vi "2_2_Face_Detection_Eval(FPGA)(PXI,sbRIO_Remote).vi"() -> ()   [LabVIEW 2020]
doc: "This example demonstrates the usage of the \"DeepLTK FPGA Addon\" for deploying a Face Detection model on a PXI-FPGA board, utilizing an input image sourced from a file.\n\nMore Examples: https://github.com/ngenehub/deepltk_fpga_examples"
uses:
  <vilib>/userDefined/High Color/nirio_resource_hc.ctl
  46bc2405-78a8-48b4-9ac8-c57804670a76.vi
  20299fb9-7878-42d1-962c-cdd5eeae2605.vi
  <vilib>/FPGAPlugInAG/Dynamic/niLvFpga_Download_Dynamic.vi
  <vilib>/FPGAPlugInAG/Dynamic/niLvFpga_Run_Dynamic.vi
  <vilib>/Ngene/Deep Learning Toolkit/Toolkit/NN_Data/subVIs/Dataset/NN_Variant_to_DVR/4D/NN_Data_Variant_to_DVR(4D_SGL).vi
  <vilib>/Ngene/Deep Learning Toolkit/Toolkit/NN_Data/subVIs/Get_Data_Vals/4D/NN_Data_Get_ValByRef(4D_SGL_idx).vi
  <vilib>/Ngene/DeepLTK FPGA Addon/Toolkit/NNF_Host/API/NNF_Set_Input/NNF_Set_Input(3D_I8).vi
  <vilib>/Ngene/Deep Learning Toolkit/Toolkit/NN_Train/Eval_Loss/NN_Eval_Test_Error_Loss/NN_Eval(In3D_OutBBox).vi
  <vilib>/Ngene/Deep Learning Toolkit/Toolkit/NN_Train/Eval_Loss/NN_Calc_Cofusion_Matrix/NN_Calc_Confusion_Matrix(In3D_OutBBox).vi
  <vilib>/FPGAPlugInAG/Dynamic/niLvFpga_Close_Dynamic.vi
  <vilib>/rvi/interface/nirviMethod/nirviMethod.xnode
  <vilib>/rvi/interface/nirviCloseFPGA/nirviCloseFPGA.xnode
  <vilib>/Ngene/Deep Learning Toolkit/Toolkit/Deep_Learning_Toolkit_by_Ngene.lvlib
  <vilib>/Ngene/DeepLTK FPGA Addon/Toolkit/DeepLTK_FPGA_Addon.lvlib
  <vilib>/ptbypt/NI_PtbyPt.lvlib
panel:
  out "Eval Time":dbl=0.030917380000028062 format="%#_2p"
  out "Loop time":dbl=0.030853959999512882 format="%#_2p"
  out "Confusion Matrix":string[][](table)=[["26", "6", "0.8125"], ["2", "0", "0.0000"], ["0.9286", "0.0000", ""]]
  out "mAP@0.5":sgl=0.788305
  out "mIOU":sgl=0.59939504
  out "Iterations":i32=19
  out "Dataset Size":i32=20
  in  "Stop":bool
  in  "FPGA Target":T1="rio://10.0.0.39/RIO0" caption="RIO Device"
  in  "FPGA Bitfile":path=path "D:/Ngene/GitHub/deepltk_fpga_examples/FPGA Bitfiles/NNF_sbRIO_9609_8Cores.lvbitx"
  in  "Dataset Path (Annotations)":path=path "D:/Ngene/GitHub/deepltk_fpga_examples/2_Face_Detection(PXI,sbRIO)/Dataset/Annotations"
  in  "Display?":bool
  out "Display":T2(plugin-control)
  in  "Scalers File Path":path=path "D:/Ngene/GitHub/deepltk_fpga_examples/2_Face_Detection(PXI,sbRIO)/Models/Face_Detection_NNF_Converted/NNF_Face_Detection_Scalers.cfg"
  in  "Dataset Path (Images)":path=path "D:/Ngene/GitHub/deepltk_fpga_examples/2_Face_Detection(PXI,sbRIO)/Dataset/Images"
  in  "Confidence_Thresh":sgl=0.46
  in  "IOU_Thresh":sgl=0.4
  in  "Weight File Path":path=path "D:/Ngene/GitHub/deepltk_fpga_examples/2_Face_Detection(PXI,sbRIO)/Models/Face_Detection_NNF_Converted/NNF_Face_Detection.bin"
  in  "Configuration File Path":path=path "D:/Ngene/GitHub/deepltk_fpga_examples/2_Face_Detection(PXI,sbRIO)/Models/Face_Detection_NNF_Converted/NNF_Face_Detection.cfg"
  # "Overview: This VI is designed to evaluate (measure the accuracy of) the model when executed on FPGA in PXI systems.\nThis VI can also be used to run the evaluation on sbRIO Targets remotely (from Windows based PC)\nRequirements: \n• DeepLTK - Deep Learning Toolkit for LabVIEW (https://www.ngene.co/deep-learning-toolkit-for-labview)\n• DeepLTK FPGA Addon (https://www.ngene.co/deepltk-accelerator-for-fpga)\nInstructions:\n1. Select FPGA target at FPGA Target control. PXI or remote sbRIO FPGA target can be specified.\n2. Provide path to compiled FPGA bitfile at FPGA Bitfile control. A sample is available in the \"Examples\\FPGA Bitfiles\" folder. \n3. Provide the path to the dataset to be evaluated at Dataset. A sample is available in the \"Dataset\" folder.\n4. Provide paths to .cfg, .bin and scalers.cfg files generated during model conversion or sample from project (locted in \"Models\\Face_Detection_NNF_Converted\" folder ) at Network Configuration File Path, Weight File Path and Scalers File Path controls.\n5. Run the VI with the default remaining settings.\n6. Observe measured accuracy at mIOU, mAP@0.5 and Confusion Matrix indicator.\n7. Press the Stop button to stop VI.\n7. To measure reference accuracy (when executed on CPU) run 2_1_Face_Detection_Eval(CPU).vi located in the project."
  # "Copy resource path from NI MAX if needed"
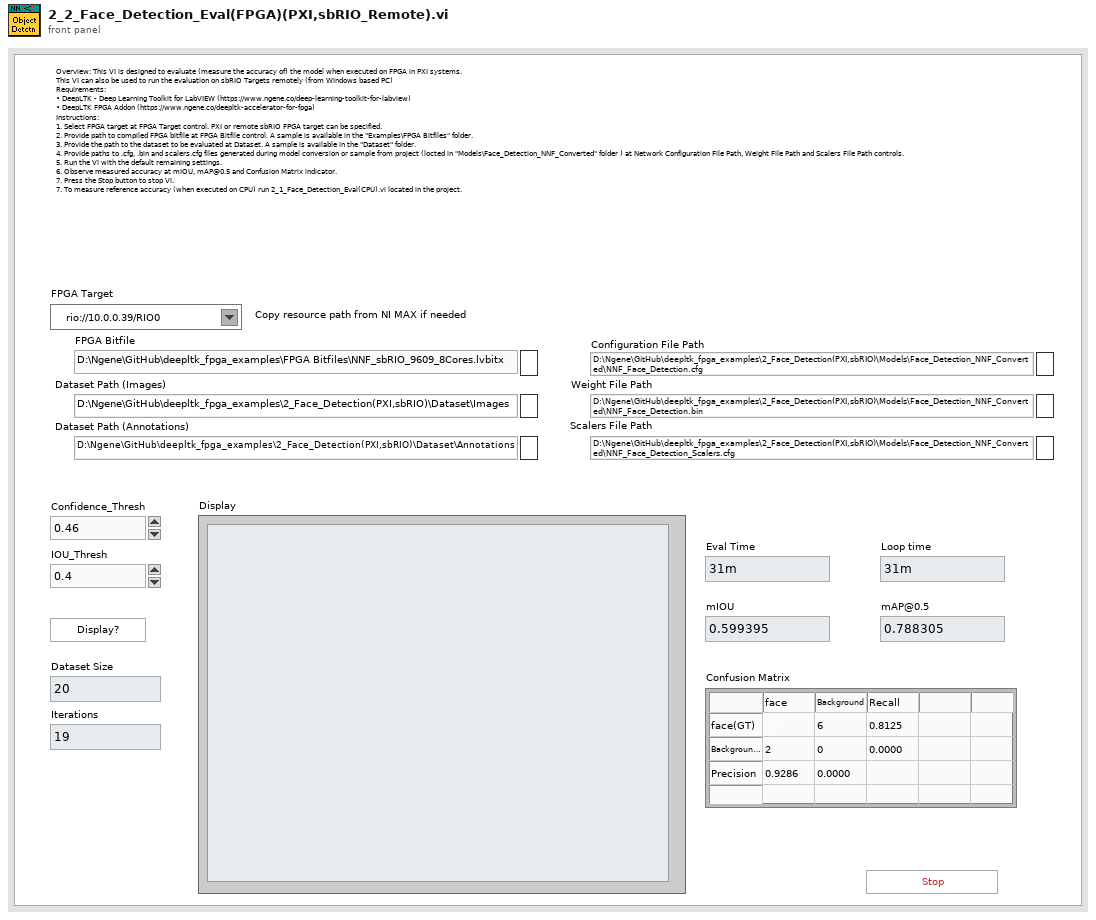
[diagram p1: front panel]
types:
  T1 = typedef "nirio_resource_hc.ctl" = tag
  T2 = typedef "IMAQ Image.ctl" = refnum<image>
  T3 = typedef "Image Type" = u32
  T4 = typedef "DeepLTK_FPGA_Addon.lvlib/NNF.ctl" = cluster{"FPGA VI Ref ":refnum<k20>, "Subnets":T5[], "Dims_In":T7, "#Cores(enum)":T8, "NN_Ref":T9}
  T5 = typedef "DeepLTK_FPGA_Addon.lvlib/NNF_Subnet.ctl" = cluster{"Subnet Type":T6, "Subnet Data":variant, "Input Scaler":sgl, "Output Scaler":sgl}
  T6 = typedef "DeepLTK_FPGA_Addon.lvlib/NNF_Subnet_Type.ctl" = enum16{"CPU", "FPGA", "Split FPGA"}
  T7 = typedef "Deep_Learning_Toolkit_by_Ngene.lvlib/NN_Dims(C,H,W).ctl" = cluster{"C":i32, "H":i32, "W":i32}
  T8 = typedef "DeepLTK_FPGA_Addon.lvlib/NNF_No_Of_Cores.ctl" = enum16{"4CH", "8CH"}
  T9 = typedef "DeepLTK_FPGA_Addon.lvlib/NN_DVR.ctl" = refnum<data-value>
  T10 = typedef "Deep_Learning_Toolkit_by_Ngene.lvlib/NN_DataSets_All(In3D_OutBBox).ctl" = cluster{"Train":T11, "Validation":T11, "Test":T11}
  T11 = typedef "Deep_Learning_Toolkit_by_Ngene.lvlib/NN_DataSet(In3D_OutBBox).ctl" = cluster{"Inputs Ref.":variant, "Dataset_Size":i32, "Dims_In":T7, "Outputs Refs":T12, "No of Classes ":i32, "Labels":string[], "File Paths":path[]}
  T12 = typedef "Deep_Learning_Toolkit_by_Ngene.lvlib/NN_Data_ref(1D_BBox).ctl" = refnum<data-value>
  T13 = typedef "Deep_Learning_Toolkit_by_Ngene.lvlib/NN_Data_ref(4D_SGL).ctl" = refnum<data-value>
  T14 = typedef "Deep_Learning_Toolkit_by_Ngene.lvlib/NN_Layer.ctl" = cluster{"Name":string, "Layer_Data":variant, "Layer_Type":T15, "Dims_In":T7, "Layers_In":variant, "Dims_Out":T7, "Layers_Out":variant, "Metrics":T16, "GPU_Data":variant, "mBatch":i32, "NN_Device":T17, "NNg_hdls":T18, "Train?":bool, "Dimty":T19, "RecptField":T20}
  T15 = typedef "Deep_Learning_Toolkit_by_Ngene.lvlib/NN_Layer_Type.ctl" = enum16{"Input1D", "Input3D", "Conv1D", "Conv2D", "Conv2D_Adv", "MaxPool", "AvgPool", "UpSample", "DropOut3D", "ShortCut", "Concat", "SoftMax3D", "FC", "DropOut", "Softmax", "Flatten", "YOLO_v2", "YOLO_v4", "Activation", "BatchNormalization", "Unsupported"}
  T16 = typedef "Deep_Learning_Toolkit_by_Ngene.lvlib/NN_Layer_Metrics.ctl" = cluster{"Data":dbl, "Params":dbl, "Ops":dbl}
  T17 = typedef "Deep_Learning_Toolkit_by_Ngene.lvlib/NN_Device.ctl" = enum16{"CPU", "GPU"}
  T18 = typedef "Deep_Learning_Toolkit_by_Ngene.lvlib/nng_cuda_handles.ctl" = cluster{"cudnn":u64, "cublas":u64, "stream":u64, "curand":u64}
  T19 = typedef "Deep_Learning_Toolkit_by_Ngene.lvlib/NN_Layer_Dimty.ctl" = enum16{"1D", "3D"}
  T20 = typedef "Deep_Learning_Toolkit_by_Ngene.lvlib/NN_Layer_RF_State.ctl" = cluster{"Dims":T21, "J":T21}
  T21 = typedef "Deep_Learning_Toolkit_by_Ngene.lvlib/NN_Dims(V,H).ctl" = cluster{"V":i32, "H":i32}
  T22 = typedef "Deep_Learning_Toolkit_by_Ngene.lvlib/NN_BBox_Detection.ctl" = cluster{"Class":i32, "Conf Level":sgl, "BBox":T23}
  T23 = typedef "Deep_Learning_Toolkit_by_Ngene.lvlib/NN_BBox.ctl" = cluster{"x":sgl, "y":sgl, "w":sgl, "h":sgl}
  T24 = typedef "Deep_Learning_Toolkit_by_Ngene.lvlib/NN.ctl" = cluster{"Name":string, "No of Layers":i32, "mBatch":i32, "Layers":T25[], "Dimty":T26, "Dims_In":T7, "Dims_Out":T7, "Working_Dir":path, "Train?":bool, "Train_Params":T27, "LR_Update_Policy":T30, "Session Data":T32, "Ground_truth":T33, "NNg_hdls":T18, "NN_Device":T17, "GPU Id":i32, "Labels":string[], "Receptive Field":T21[], "Loss_Type":T34, "Loss_Cfg_Prms":variant, "NNG_WS":T35}
  T25 = typedef "Deep_Learning_Toolkit_by_Ngene.lvlib/NN_Layer_ref.ctl" = refnum<data-value>
  T26 = typedef "Deep_Learning_Toolkit_by_Ngene.lvlib/NN_In_Out_Dim-ty.ctl" = enum8{"In1D_Out1D", "In3D_Out1D", "In3D_Out3D", "In3D_OutBBox"}
  T27 = typedef "Deep_Learning_Toolkit_by_Ngene.lvlib/NN_Train_Params.ctl" = cluster{"Optimizer":T28, "Beta_1":sgl, "Beta_2":sgl, "Weight Decay(L1)":sgl, "Weight Decay(L2)":sgl, "Data_Sampling":T29}
  T28 = typedef "Deep_Learning_Toolkit_by_Ngene.lvlib/NN_Train_Optimizer.ctl" = enum16{"SGD", "Adam", "Adagrad", "Adadelta", "RMSProp", "Nesterov"}
  T29 = typedef "Deep_Learning_Toolkit_by_Ngene.lvlib/NN_Train_Data_Sampling.ctl" = enum16{"Random", "Sequential"}
  T30 = typedef "Deep_Learning_Toolkit_by_Ngene.lvlib/NN_LR_Policy_Cfg.ctl" = cluster{"Policy_Type":T31, "LR0":dbl, "k":sgl, "WarmUp_Policy":enum16{"Step", "Ramp"}, "WarmUp_Iter":i32, "WarmUp_Ratio":sgl}
  T31 = typedef "Deep_Learning_Toolkit_by_Ngene.lvlib/NN_LR_Policy_Type.ctl" = enum16{"Manual", "Step", "Exp", "1/t"}
  T32 = typedef "Deep_Learning_Toolkit_by_Ngene.lvlib/NN_Train_Session_Data.ctl" = cluster{"Epochs":sgl, "Tot_Iter":i32, "LR":sgl, "LR_iter":i32}
  T33 = typedef "Deep_Learning_Toolkit_by_Ngene.lvlib/NN_Ground_truth.ctl" = cluster{"Y":variant}
  T34 = typedef "Deep_Learning_Toolkit_by_Ngene.lvlib/NN_Loss_Type.ctl" = enum16{"None", "MSE", "CrossEntropy", "YOLO_v2", "YOLO_v4"}
  T35 = typedef "Deep_Learning_Toolkit_by_Ngene.lvlib/NNG_WS.ctl" = cluster{"NNG_WS_Mem":T36, "Max_WS_Size":i64}
  T36 = typedef "Deep_Learning_Toolkit_by_Ngene.lvlib/NNg_WS_Mem_DVR.ctl" = refnum<data-value>
  T37 = typedef "Deep_Learning_Toolkit_by_Ngene.lvlib/NN_Eval_Params(in3D_OutBBox).ctl" = cluster{"Precision@Max_Avg_F1_Score":sgl, "Recall@Max_Avg_F1_Score":sgl, "argmax_avgF1_Score(Conf)":sgl, "Max_Avg_F1_Score":sgl, "Max_F1_Score_Per_Class":sgl[], "F1_Score_Per_Class":sgl[][], "Avg_F1,P,R Curves":cluster{"Conf":sgl[], "F1|P|R":sgl[]}[], "mIOU":sgl, "APs@0.5":sgl[], "PR_Curves@0.5":T38, "IOUs":sgl[], "mAP@0.75":sgl, "mAP@0.5-0.95":sgl, "mAP@0.5":sgl, "Mean_PR_Curve":T39}
  T38 = typedef "Deep_Learning_Toolkit_by_Ngene.lvlib/NN_PR_Curves.ctl" = T39[]
  T39 = typedef "Deep_Learning_Toolkit_by_Ngene.lvlib/NN_PR.ctl" = cluster{"Recall":sgl[], "Precision":sgl[]}
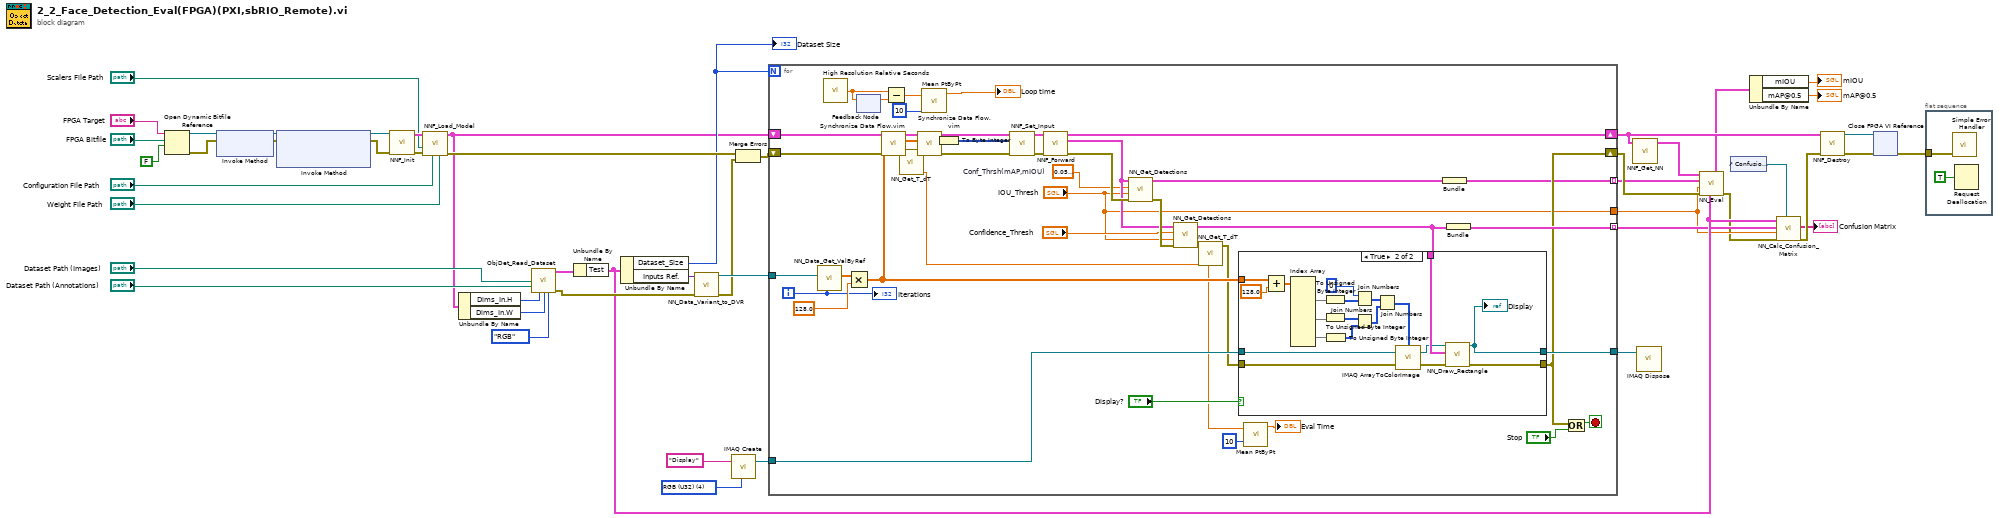
[diagram p0: block diagram]
diagram:
  w47 = T3 4 items=["Grayscale (U8)", "Grayscale (I16)", "Grayscale (SGL)", "Complex (CSG)", "RGB (U32)", "HSL (U32)", "RGB (U64)", "Grayscale (U16)"] ("Image Type")
  n1 = Open Dynamic Bitfile Reference(0:"FPGA Target", 1:"FPGA Bitfile", 2:FALSE ("Run When Loaded")) -> (5:w45:refnum<k20>, 8:w41:errorcluster)  [unwired: 2 in]
  n2 = xnode "Invoke Method"("FPGA VI Reference In"=w45, "error in"=w41) -> ("FPGA VI Reference Out"=w42:refnum<k20>, "error out"=w39:errorcluster)
  n3 = xnode "Invoke Method"("FPGA VI Reference In"=w42, "error in"=w39) -> ("FPGA VI Reference Out"=w40:refnum<k20>, "error out"=w38:errorcluster)  [unwired: 1 in]
  n4 = call <vilib>:"NNF_Init.vi"("error in"=w38, "FPGA Interface"=w40) -> ("error out"=w46:errorcluster, "NNF out"=w44:T4)  [unwired: 7 in, 1 out]
  n5 = call <vilib>:"NNF_Load_Model.vi"("Weight File Path"="Weight File Path", "Network CFG File Path"="Configuration File Path", "Error in"=w46, "Scalers"="Scalers File Path", "NNF in"=w44) -> ("error Out"=w37:errorcluster, "NNF out"=w4:T4)  [unwired: 5 in]
  n6 = Unbundle By Name(w4) -> ("Dims_In.H"=w3:i32, "Dims_In.W"=w2:i32)
  n7 = call "ObjDet_Read_Dataset.vi"("Image Path(Test)"="Dataset Path (Images)", "Anno Path(Test)"="Dataset Path (Annotations)", "Img Height"=w3, "Img Width"=w2, "Img Type"=enum16{"Grayscale", "RGB"}."RGB") -> ("Dataset"=w31:T10, "error out"=w18:errorcluster)  [unwired: 7 in, 2 out]
  n8 = Unbundle By Name(w31) -> ("Test"=w13:T11)
  n9 = Unbundle By Name(w13) -> ("Dataset_Size"=w14:i32, "Inputs Ref."=w30:variant)
  "Dataset Size" <- w14
  n10 = call-poly <vilib>:"NN_Data_Variant_to_DVR.vi"("error in (no error)"=w18, "Inputs Ref."=w30) -> ("error out"=w16:errorcluster, "DVR(4D_SGL)"=w29:T13)  [unwired: 8 in]
  n11 = call "IMAQ Create"("Image Name"="Display", "Image Type"=w47) -> ("New Image"=w48:T2)  [unwired: 3 in, 1 out]
  n12 = Merge Errors(w37, w16) -> (w17:errorcluster)
  n13 = for {
    N: w14 -> [_]
    shift-right: [w92] -> w26
    shift-left: w4 -> [w74]
    tunnel: w48 -> [w85]
    shift-right: [w79] -> w23
    shift-left: w17 -> [w72]
    tunnel: w29 -> [w88]
    tunnel: [w84] -> w12 mode=indexing
    tunnel: [w83] -> w27
    tunnel: ["IOU_Thresh"] -> w11
    tunnel: [w52] -> w1 mode=indexing
    i -> [w76]
    stop <- w78 stop-if-true
    w56 = sgl 0.05  # Conf_Thrsh(mAP,mIOU)
    # "Inference Loop"
    n14 = call-poly <vilib>:"NN_Data_Get_ValByRef.vi"("index (vol)"=w76, "DVR(4D_SGL)"=w88) -> ("Value(3D_SGL)"=w90:sgl[][][])  [unwired: 6 in, 1 out]
    n15 = call <vilib>:"High Resolution Relative Seconds.vi"() -> ("relative seconds"=w81:dbl)
    n16 = Multiply(x=w90, y=sgl 128.0 ("x")) -> (x*y=w73:sgl[][][])
    n17 = feedback-in #1(w81) -> ()
    n18 = feedback #1() -> (w82:dbl)  [unwired: 1 in]
    n19 = call "Synchronize Data Flow.vim"("input 4"=w72, "input 2"=w73, "input 1"=w74) -> ("output 4"=w69:errorcluster, "output 2"=w70:sgl[][][], "output 1"=w71:T4)  [unwired: 1 in, 1 out]
    n20 = Subtract(x=w81, y=w82) -> (x-y=w80:dbl)
    n21 = call <vilib>:"NN_Get_T_dT.vi"("error in (no error)"=w69) -> ("T_out"=w58:dbl, "error out"=w65:errorcluster)  [unwired: 6 in, 1 out]
    n22 = call "Synchronize Data Flow.vim"("input 4"=w65, "input 2"=w70, "input 1"=w71) -> ("output 4"=w66:errorcluster, "output 2"=w68:sgl[][][], "output 1"=w67:T4)  [unwired: 1 in, 1 out]
    n23 = call <vilib>:"Mean PtByPt.vi"("x"=w80, "sample length"=10) -> ("mean"=→"Loop time":dbl)  [unwired: 2 in, 1 out]
    n24 = To Byte Integer(number=w68) -> (8bit integer=w87:i8[][][])
    n25 = call-poly <vilib>:"NNF_Set_Input.vi"("error in"=w66, "Data_in(3D_I8)"=w87, "NNF in"=w67) -> ("error out"=w93:errorcluster, "NNF out"=w94:T4)  [unwired: 7 in]
    n26 = call <vilib>:"NNF_Forward.vi"("error in"=w93, "NNF in"=w94) -> ("error out"=w91:errorcluster, "Last_Layer"=w57:T14, "NNF out"=w92:T4)  [unwired: 7 in]
    n27 = call <vilib>:"NN_Get_Detections.vi"("error in"=w91, "IOU_Thrsh"="IOU_Thresh", "Confidence_Thrsh"=w56, "YOLO_Layer"=w57) -> ("error out"=w63:errorcluster, "Detections"=w53:T22[])  [unwired: 6 in]
    n28 = call <vilib>:"NN_Get_Detections.vi"("error in"=w63, "IOU_Thrsh"="IOU_Thresh", "Confidence_Thrsh"="Confidence_Thresh", "YOLO_Layer"=w57) -> ("error out"=w62:errorcluster, "Detections"=w54:T22[])  [unwired: 6 in]
    n29 = call <vilib>:"NN_Get_T_dT.vi"("T_in"=w58, "error in (no error)"=w62) -> ("error out"=w61:errorcluster, "dT"=w59:dbl)  [unwired: 5 in, 1 out]
    n30 = case shown="True" "Display?" {
      tunnel: w61 -> [w96 w116]
      tunnel: w85 -> [w95 w115]
      tunnel: w54 -> [_ w105]
      tunnel: [w96 w102] -> w79
      tunnel: w73 -> [_ w101]
      tunnel: [w95 w97] -> w83
      frame False {
      }
      frame True {
        n31 = Add(x=w101, y=sgl 128.0 ("x")) -> (x+y=w103:sgl[][][])
        n32 = Index Array(array=w103) -> (element #1=w114:sgl[][], element #2=w111:sgl[][], element #3=w109:sgl[][])  [unwired: 9 in]
        n33 = To Unsigned Byte Integer(number=w114) -> (unsigned 8bit integer=w113:u8[][])
        n34 = To Unsigned Byte Integer(number=w111) -> (unsigned 8bit integer=w110:u8[][])
        n35 = To Unsigned Byte Integer(number=w109) -> (unsigned 8bit integer=w108:u8[][])
        n36 = Join Numbers(hi=u8 0, lo=w113) -> ((hi.lo)=w112:u16[][])
        n37 = Join Numbers(hi=w110, lo=w108) -> ((hi.lo)=w107:u16[][])
        n38 = Join Numbers(hi=w112, lo=w107) -> ((hi.lo)=w100:u32[][])
        n39 = call "IMAQ ArrayToColorImage"("Image Pixels (U32)"=w100, "Image"=w115, "error in (no error)"=w116) -> ("Image Out"=w104:T2, "error out"=w98:errorcluster)  [unwired: 2 in]
        n40 = call "NN_Draw_Rectangle.vi"("error in (no error)"=w98, "Draw_Boxes"=w105, "Image_in"=w104) -> ("error out"=w102:errorcluster, "Image_out"=w97:T2)  [unwired: 6 in, 1 out]
        "Display" <- w97
      }
    }
    n41 = call <vilib>:"Mean PtByPt.vi"("x"=w59, "sample length"=10) -> ("mean"=→"Eval Time":dbl)  [unwired: 2 in, 1 out]
    n42 = Bundle("Detections"=w53) -> (w52:cluster{"Detections":T22[]})  [unwired: 1 in]
    n43 = Bundle("Detections"=w54) -> (w84:cluster{"Detections":T22[]})  [unwired: 1 in]
    n44 = Or(x=w79, y="Stop") -> (x .or. y?=w78:bool)
    "Iterations" <- w76
  }
  n45 = call "NNF_Get_NN.vi"("NNF in"=w26) -> ("NN out"=w25:T24)  [unwired: 10 in]
  n46 = call "IMAQ Dispose"("Image"=w27) -> ()  [unwired: 5 in, 1 out]
  n47 = call-poly <vilib>:"NN_Eval.vi"("Dataset"=w13, "error in"=w23, "IOU_Conf_Thrsh(0.5)"=w11, "Detections(in Dataset)"=w1, "NN in"=w25) -> ("error out"=w10:errorcluster, "NN_Eval_Params"=w24:T37)  [unwired: 4 in, 1 out]
  n48 = control-ref of="Confusion Matrix"() -> (w7:refnum<vi>)
  n49 = Unbundle By Name(w24) -> ("mIOU"=→"mIOU":sgl, "mAP@0.5"=→"mAP@0.5":sgl)
  n50 = call-poly <vilib>:"NN_Calc_Confusion_Matrix.vi"("Confusion Matrix (Table) ref."=w7, "error in (no error)"=w10, "TP_IOU_Thrsh(0.5)"=w11, "Predictions"=w12, "Dataset"=w13) -> ("error out"=w9:errorcluster, "Confusion Matrix (Table)"=→"Confusion Matrix":string[][])  [unwired: 3 in, 2 out]
  n51 = call <vilib>:"NNF_Destroy.vi"("error in"=w9, "NNF in"=w26) -> ("error out"=w36:errorcluster, "FPGA VI Ref"=w34:refnum<k20>)  [unwired: 8 in]
  n52 = xnode "Close FPGA VI Reference"("FPGA VI Reference In"=w34, "error in"=w36) -> ("error out"=w35:errorcluster)
  n53 = flat-sequence {
    tunnel: w35 -> [w117]
    frame #0 {
      n54 = call <vilib>:"Simple Error Handler.vi"("error in (no error)"=w117) -> ()  [unwired: 4 in, 5 out]
      n55 = Request Deallocation(TRUE ("flag")) -> ()
    }
  }
